vi "add channel to configuration dialog launcher.vi"(5 "channels":refnum<vi>, 7 "user event":T1, 8 "error in":errorcluster, 10 "engine configuration.lvclass in":refnum<class "engine configuration.lvclass">, 11 "Scan Engine configuration in":refnum<class "Scan Engine configuration.lvclass">) -> (0 "error out":errorcluster, 2 "engine configuration.lvclass out":refnum<class "engine configuration.lvclass">, 3 "Scan Engine configuration out":refnum<class "Scan Engine configuration.lvclass">)   [LabVIEW 2013, in "Scan Engine editor node.lvclass"]
uses:
  Scan Engine editor node.lvclass
  <vilib>/NI/Module Execution Interface/Engine Configuration/engine configuration.lvclass
  module/configuration/Scan Engine configuration.lvclass
  <vilib>/NI/Configuration Framework/Node/UserEventRef.ctl
  <vilib>/NI/Configuration Framework/Controls/EventCluster.ctl
  <vilib>/NI/Configuration Framework/serializable configuration/NISE_CEF_serializable configuration.lvclass/NISE_CEF_serializable configuration.ctl
  <vilib>/NI/Tag Bus/tag/tag descriptor.lvclass/tag descriptor.ctl
  <vilib>/NI/Tag Bus/tag/write tag name.vi
  <vilib>/Utility/LVClass/Get LV Class Name.vi
  <vilib>/NI/Configuration Framework/error generator/NISE_error generator.vi
  <vilib>/NI/Configuration Framework/NISE_CEF_TreeControl.lvlib
  <vilib>/NI/Tag Bus Module Framework/channel/TBM channel.lvclass
  <vilib>/NI/Configuration Framework/serializable configuration/NISE_CEF_serializable configuration.lvclass
  <vilib>/NI/Configuration Framework/Node/NISE_CEF_Node.lvclass
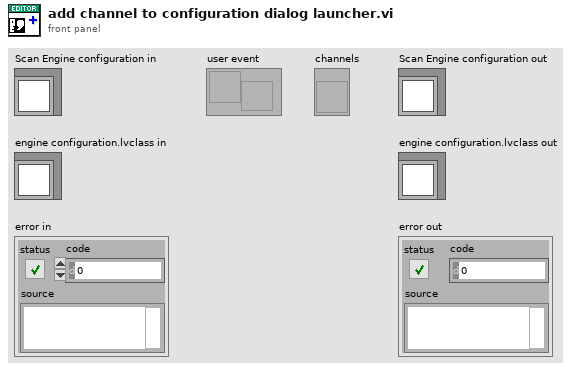
[diagram p1: front panel]
types:
  T1 = typedef "NISE_CEF_Node.lvclass/UserEventRef.ctl" = refnum<user-event>
  T2 = typedef "Scan Engine editor node.lvclass/table line.ctl" = cluster{"tag":string, "channel":refnum<class "TBM channel.lvclass">}
  T3 = typedef "NISE_CEF_TreeControl.lvlib/EventCluster.ctl" = cluster{"command":string, "data":string}
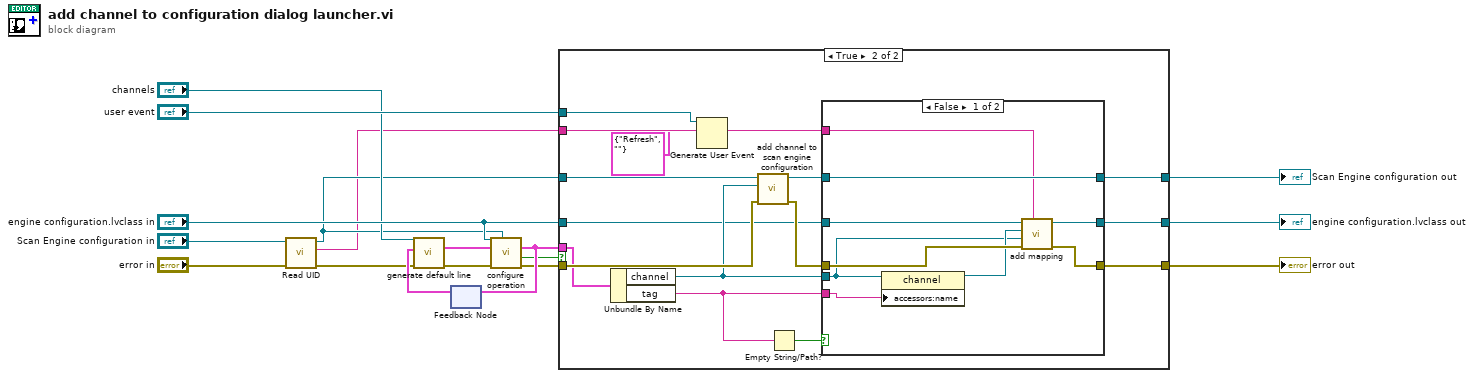
[diagram p0: block diagram]
diagram:
  n1 = call <vilib>:"Read UID.vi"("error in"="error in", "configuration in"="Scan Engine configuration in") -> ("error out"=w4:errorcluster, "instance id"=w1:string, "configuration out"=w2:refnum<class "Scan Engine configuration.lvclass">)  [unwired: 7 in]
  n2 = feedback #1() -> (w17:T2)  [unwired: 1 in]
  n3 = call "generate default line.vi"("error in"=w4, "last line item"=w17, "operations table"="channels") -> ("error out"=w8:errorcluster, "line item in"=w11:T2)  [unwired: 7 in]
  n4 = call "configure operation.vi"("Scan Engine configuration"=w2, "error in"=w8, "line item in"=w11, "engine configuration in"="engine configuration.lvclass in") -> ("error out"=w7:errorcluster, "success"=w9:bool, "line item out"=w16:T2)  [unwired: 4 in, 1 out]
  n5 = feedback-in #1(w16) -> ()
  n6 = case shown="True" w9 {
    tunnel: [w20 w25] -> w5
    tunnel: [w19 w24] -> w14
    tunnel: w7 -> [w20 w32]
    tunnel: "engine configuration.lvclass in" -> [w18 w29]
    tunnel: w16 -> [_ w31]
    tunnel: w1 -> [_ w35]
    tunnel: w2 -> [w19 w34]
    tunnel: [w18 w26] -> w15
    tunnel: "user event" -> [_ w21]
    frame False {
    }
    frame True {
      n7 = Unbundle By Name(w31) -> ("channel"=w30:refnum<class "TBM channel.lvclass">, "tag"=w28:string)
      n8 = Generate User Event(user event=w21, event data cluster=T3 {"command"="Refresh", "data"=""} ("event data")) -> ()  [unwired: 2 in, 2 out]
      n9 = call "add channel to scan engine configuration.vi"("error in"=w32, "channel"=w30, "Scan Engine configuration in"=w34) -> ("error out"=w33:errorcluster, "Scan Engine configuration out"=w23:refnum<class "Scan Engine configuration.lvclass">)  [unwired: 7 in]
      n10 = Empty String/Path?(string/path=w28) -> (empty?=w27:bool)
      n11 = case shown="False" w27 {
        tunnel: w33 -> [w44 w47]
        tunnel: [w43 w47] -> w25
        tunnel: w35 -> [w36 _]
        tunnel: w30 -> [w39 _]
        tunnel: w28 -> [w42 _]
        tunnel: w29 -> [w40 w46]
        tunnel: [w38 w46] -> w26
        tunnel: [w37 w45] -> w24
        tunnel: w23 -> [w37 w45]
        frame False {
          n12 = property class="channel"(reference=w39, "accessors:name"=w42) -> (reference out=w41:refnum<class "TBM channel.lvclass">)  [unwired: 1 in, 1 out]
          n13 = call <vilib>:"add mapping.vi"("owner ID"=w36, "error in"=w44, "channel"=w39, "tag descriptor"=w41, "engine configuration"=w40) -> ("error out"=w43:errorcluster, "engine configuration out"=w38:refnum<class "engine configuration.lvclass">)  [unwired: 5 in]
        }
        frame True {
        }
      }
    }
  }
  "engine configuration.lvclass out" <- w15
  "Scan Engine configuration out" <- w14
  "error out" <- w5
